vi "Save VI.vi"(8 "error in (no error)":errorcluster, 11 "VI in":refnum<class "VI.lvclass">) -> (0 "error out":errorcluster, 3 "VI out":refnum<class "VI.lvclass">)   [LabVIEW 2025, in "VI.lvclass"]
doc: "Save the autogenerated FPGA VI."
uses:
  VI.lvclass
  VI.lvclass/VI.ctl
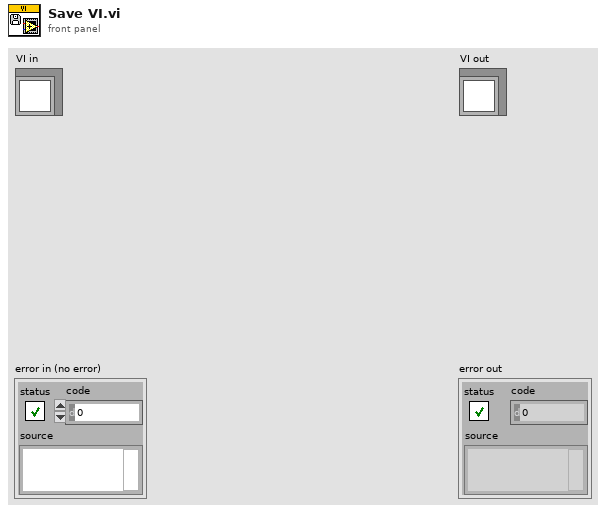
[diagram p1: front panel]
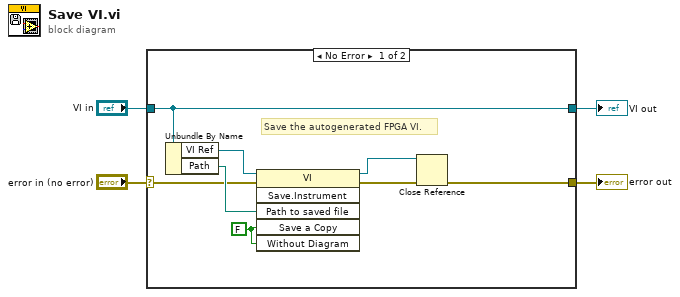
[diagram p0: block diagram]
diagram:
  n1 = case shown="No Error" "error in (no error)" {
    selector: "error in (no error)" -> [w8 w14]
    tunnel: [w6 w14] -> w3
    tunnel: [w12 w13] -> w1
    tunnel: "VI in" -> [w12 w13]
    frame No Error {
      w9 = FALSE ("Save a Copy")
      # "Save the autogenerated FPGA VI."
      n2 = Unbundle By Name(w12) -> ("VI Ref"=w11:refnum<vi>, "Path"=w10:path)
      n3 = invoke class="VI" method="Save.Instrument"(reference=w11, error in=w8, "Path to saved file"=w10, "Save a Copy"=w9, "Without Diagram"=w9) -> (reference out=w5:refnum<vi>, error out=w7:errorcluster)  [unwired: 1 in, 4 out]
      n4 = Close Reference(reference=w5, error in (no error)=w7) -> (error out=w6:errorcluster)
    }
    frame Error {
    }
  }
  "error out" <- w3
  "VI out" <- w1
